vi "CAN Komm.vi"(8 "error in":errorcluster) -> (0 "error out":errorcluster)   [LabVIEW 2020, in "CAN Interface.lvlib"]
uses:
  CAN Interface.lvlib
  CAN Komm Aktionen.ctl
  FGV CAN Daten Aktionen.ctl
  <vilib>/xnet/xnet.llb/XNET CAN Comm State.ctl
  <vilib>/xnet/xnet.llb/XNET Control Scope.ctl
  <vilib>/xnet/xnet.llb/XNET Create Session (Frame Output Stream).vi
  <vilib>/xnet/xnet.llb/XNET Write (Frame CAN).vi
  <vilib>/xnet/xnet.llb/XNET Read (State CAN Comm).vi
  <vilib>/xnet/xnet.llb/XNET Create Session (Frame Input Stream).vi
  <vilib>/xnet/xnet.llb/XNET Read (Frame CAN).vi
  <resource>/objmgr/xnet.rc
  Allgemein/Allgemein.lvlib
panel:
  in  "interface":refnum<k21>="CAN1"
  in  "cluster (:memory:)":refnum<k21>="nixnet_example.CAN_Cluster"
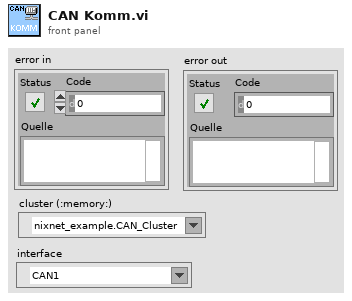
[diagram p1: front panel]
types:
  T1 = typedef "CAN Interface.lvlib/CAN Komm Aktionen.ctl" = enum16{"lesen", "init", "Komm", "beenden", "flush"}
  T2 = typedef "CAN Interface.lvlib/FGV CAN Daten Aktionen.ctl" = enum16{"lesen", "Daten", "Konfig", "laden", "speichern", "Status"}
  T3 = typedef "XNET CAN Comm State.ctl" = u8
  T4 = typedef "CAN Konfig.lvlib/Konfig Daten PC.ctl" = cluster{"Baude Rate":T5, "COM state":u8, "Frame-ID FTIR Start":u32, "Frame-ID FTIR End":u32, "Frame-ID Status Start":u32, "Frame-ID Status End":u32, "Zustand Information":u32, "Aktion":u32, "Frame-ID FTIR Arry":u32[], "Frame-ID Status Arry":u32[], "GPS Start":u32, "Interface":refnum<k21>}
  T5 = typedef "CAN Interface.lvlib/Baude Rate.ctl" = u32
  T6 = typedef "XNET Frame CAN.ctl" = cluster{"timestamp":timestamp, "payload":u8[], "identifier":u32, "type":T7, "extended?":bool, "echo?":bool}
  T7 = typedef "XNET Frame Type CAN.ctl" = u8
  T8 = typedef "XNET Control Scope.ctl" = u32
  T9 = typedef "XNET CAN Comm.ctl" = cluster{"fault code":i32, "fault?":bool, "communication state":T3, "last error":T10, "receive error counter":u8, "transmit error counter":u8, "transceiver error?":bool, "sleep?":bool}
  T10 = typedef "XNET CAN Last Err.ctl" = u8
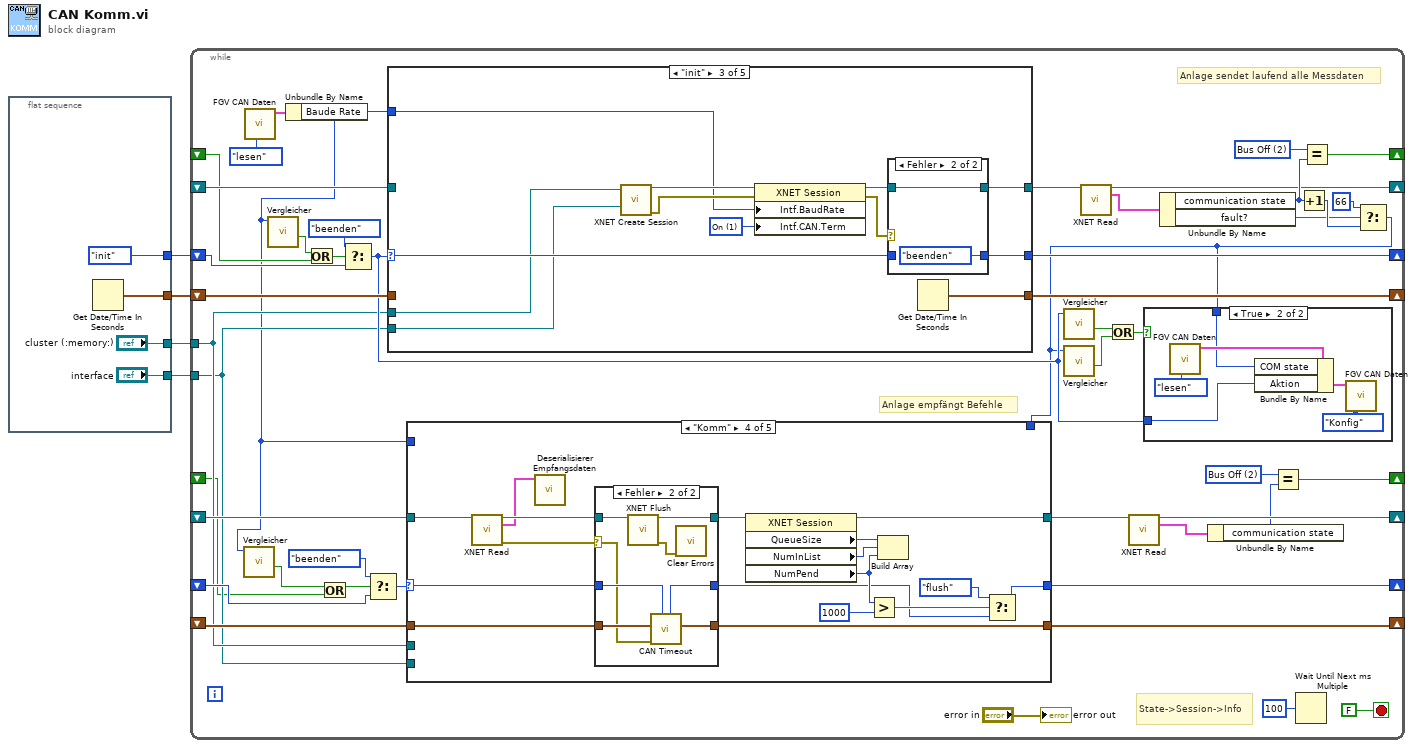
[diagram p0: block diagram]
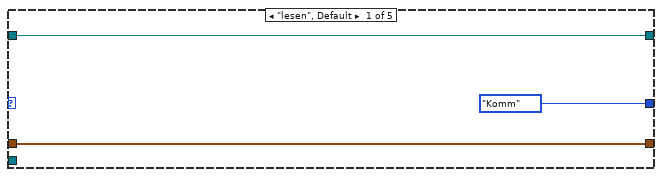
[diagram p3: hidden frame]
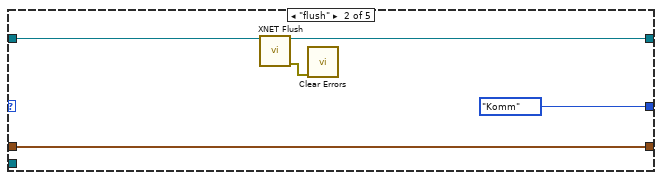
[diagram p4: hidden frame]
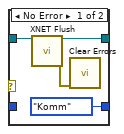
[diagram p5: hidden frame]
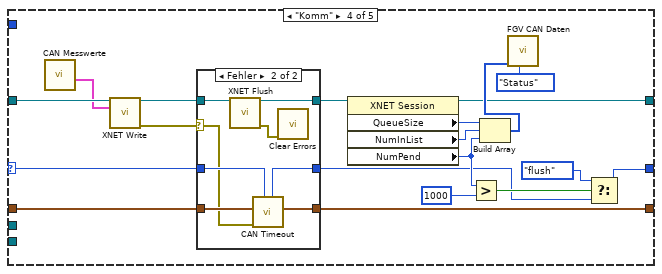
[diagram p6: hidden frame]
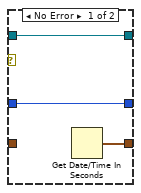
[diagram p7: hidden frame]
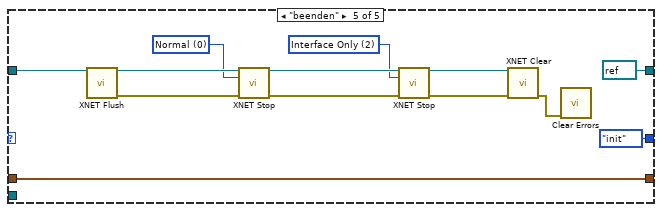
[diagram p8: hidden frame]
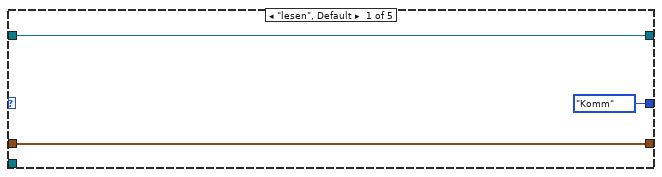
[diagram p9: hidden frame]
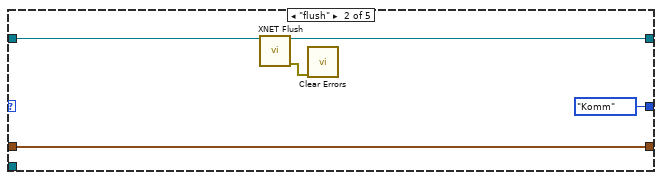
[diagram p10: hidden frame]
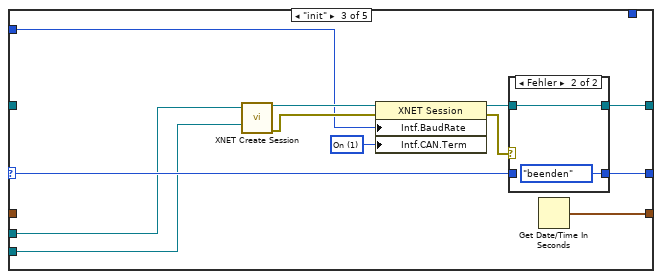
[diagram p11: hidden frame]
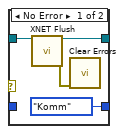
[diagram p12: hidden frame]
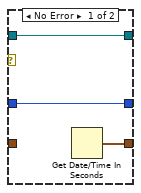
[diagram p13: hidden frame]
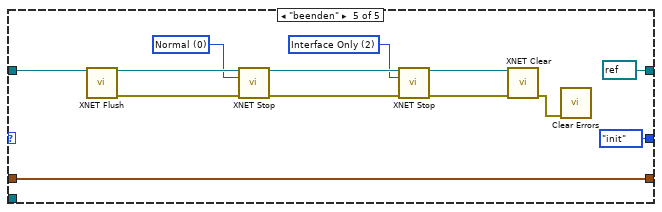
[diagram p14: hidden frame]
diagram:
  n1 = flat-sequence {
    tunnel: [CAN_Komm_Aktionen."init" ("Aktionen")] -> w4
    tunnel: [w7] -> w3
    tunnel: ["cluster (:memory:)"] -> w2
    tunnel: ["interface"] -> w1
    frame #0 {
      n2 = Get Date/Time In Seconds() -> (seconds since 1Jan1904=w7:timestamp)
    }
  }
  n3 = while {
    shift-right: [w14] -> _
    shift-left: _ -> [w55]
    shift-right: [w51] -> _
    shift-left: w4 -> [w48]
    shift-right: [w53] -> _
    shift-left: w3 -> [w54]
    tunnel: w2 -> [w23]
    tunnel: w1 -> [w22]
    shift-right: [w12] -> _
    shift-left: _ -> [w31]
    shift-right: [w20] -> _
    shift-left: _ -> [w28]
    shift-right: [w27] -> _
    shift-left: _ -> [w26]
    shift-right: [w25] -> _
    shift-left: _ -> [w24]
    shift-right: [w13] -> _
    shift-left: _ -> [w15]
    stop <- FALSE stop-if-true
    w18 = T3 2 items=["Error Active", "Error Passive", "Bus Off", "Init"] ("x")
    w33 = T3 2 items=["Error Active", "Error Passive", "Bus Off", "Init"] ("x")
    # "Anlage empfängt Befehle"
    # "Anlage sendet laufend alle Messdaten"
    # "State->Session->Info"
    n4 = call "FGV CAN Daten.vi"("Aktionen"=FGV_CAN_Daten_Aktionen."lesen") -> ("Konfig Daten"=w50:T4)  [unwired: 8 in, 2 out]
    n5 = Unbundle By Name(w50) -> ("Baude Rate"=w10:T5)
    n6 = call "Vergleicher.vi"("Numerisch"=w10) -> ("Änderung"=w30:bool)  [unwired: 10 in]
    n7 = call "Vergleicher.vi"("Numerisch"=w10) -> ("Änderung"=w46:bool)  [unwired: 10 in]
    n8 = Or(x=w46, y=w31) -> (x .or. y?=w32:bool)
    n9 = Or(x=w30, y=w15) -> (x .or. y?=w16:bool)
    n10 = Select(t=CAN_Komm_Aktionen."beenden" ("Aktionen"), s=w32, f=w48) -> (s? t:f=w44:T1)
    n11 = Select(t=CAN_Komm_Aktionen."beenden" ("Aktionen"), s=w16, f=w26) -> (s? t:f=w9:T1)
    n12 = case shown="\"init\"" w44 {
      selector: w44 -> [_ _ w78 w103 _]
      tunnel: w55 -> [w64 w66 _ w106 w128]
      tunnel: [w64 w65 w73 w89 refnum<k21> refnum ("session out")] -> w45
      tunnel: [CAN_Komm_Aktionen."Komm" ("Aktionen") CAN_Komm_Aktionen."Komm" ("Aktionen") w77 w92 CAN_Komm_Aktionen."init" ("Aktionen")] -> w51
      tunnel: w54 -> [w62 w68 _ w104 w129]
      tunnel: [w62 w68 w76 w105 w129] -> w53
      tunnel: w10 -> [_ _ w72 _ _]
      tunnel: w23 -> [_ _ w71 _ _]
      tunnel: w22 -> [_ _ w70 _ _]
      frame "lesen", Default {
      }
      frame "flush" {
        n13 = call <vilib>:"XNET Flush.vi"("session in"=w66) -> ("session out"=w65:refnum<k21>, "error out"=w67:errorcluster)  [unwired: 13 in]
        n14 = call <vilib>:"Clear Errors.vi"("error in (no error)"=w67) -> ()  [unwired: 5 in, 2 out]
      }
      frame "init" {
        w79 = u32 1 items=["Off", "On"] ("Interface:CAN:Termination")
        n15 = call-poly <vilib>:"XNET Create Session.vi"("cluster (:memory:)"=w71, "interface"=w70) -> ("session out"=w80:refnum<k21>, "error out"=w81:errorcluster)  [unwired: 12 in]
        n16 = property class="XNET Session"(reference=w80, error in=w81, "Intf.BaudRate"=w72, "Intf.CAN.Term"=w79) -> (reference out=w74:refnum<k21>, error out=w75:errorcluster)
        n17 = case shown="Fehler" w75 {
          tunnel: w78 -> [_ _]
          tunnel: [CAN_Komm_Aktionen."Komm" ("Aktionen") CAN_Komm_Aktionen."beenden" ("Aktionen")] -> w77
          tunnel: w74 -> [w84 w87]
          tunnel: [w83 w87] -> w73
          frame No Error {
            n18 = call <vilib>:"XNET Flush.vi"("session in"=w84) -> ("session out"=w83:refnum<k21>, "error out"=w82:errorcluster)  [unwired: 13 in]
            n19 = call <vilib>:"Clear Errors.vi"("error in (no error)"=w82) -> ()  [unwired: 5 in, 2 out]
          }
          frame Error {
          }
        }
        n20 = Get Date/Time In Seconds() -> (seconds since 1Jan1904=w76:timestamp)
      }
      frame "Komm" {
        n21 = call "CAN Messwerte.vi"() -> ("CAN data"=w88:T6[])  [unwired: 11 in]
        n22 = call-poly <vilib>:"XNET Write.vi"("session in"=w106, "data"=w88) -> ("session out"=w90:refnum<k21>, "error out"=w102:errorcluster)  [unwired: 1 in, 11 out]
        n23 = case shown="Fehler" w102 {
          selector: w102 -> [_ w113]
          tunnel: [w109 w116] -> w105
          tunnel: w104 -> [_ w117]
          tunnel: w103 -> [w108 w115]
          tunnel: [w108 w114] -> w93
          tunnel: w90 -> [w107 w112]
          tunnel: [w107 w111] -> w101
          frame No Error {
            n24 = Get Date/Time In Seconds() -> (seconds since 1Jan1904=w109:timestamp)
          }
          frame Error {
            n25 = call <vilib>:"XNET Flush.vi"("session in"=w112) -> ("session out"=w111:refnum<k21>, "error out"=w110:errorcluster)  [unwired: 13 in]
            n26 = call "CAN Timeout.vi"("Aktionen"=w115, "Fehler"=w113, "Zeitstempel"=w117) -> ("Zeitstempel"=w116:timestamp, "Aktionen"=w114:T1)  [unwired: 7 in]
            n27 = call <vilib>:"Clear Errors.vi"("error in (no error)"=w110) -> ()  [unwired: 5 in, 2 out]
          }
        }
        n28 = property class="XNET Session"(reference=w101) -> (reference out=w89:refnum<k21>, "QueueSize"=w99:u32, "NumInList"=w98:u32, "NumPend"=w96:u32)  [unwired: 1 in, 1 out]
        n29 = Greater?(x=w96, y=u32 1000) -> (0:w94:bool)
        n30 = Build Array(w99, w98, w96) -> (w97:u32[])
        n31 = call "FGV CAN Daten.vi"("Aktionen"=FGV_CAN_Daten_Aktionen."Status", "Status"=w97) -> ()  [unwired: 7 in, 3 out]
        n32 = Select(t=CAN_Komm_Aktionen."flush", s=w94, f=w93) -> (s? t:f=w92:T1)
      }
      frame "beenden" {
        w121 = T8 2 items=["Normal", "Session Only", "Interface Only", "Session Only Blocking"] ("scope (normal)")
        w124 = T8 0 items=["Normal", "Session Only", "Interface Only", "Session Only Blocking"] ("scope (normal)")
        n33 = call <vilib>:"XNET Flush.vi"("session in"=w128) -> ("session out"=w127:refnum<k21>, "error out"=w126:errorcluster)  [unwired: 13 in]
        n34 = call <vilib>:"XNET Stop.vi"("session in"=w127, "scope (normal)"=w124, "error in (no error)"=w126) -> ("session out"=w123:refnum<k21>, "error out"=w122:errorcluster)  [unwired: 11 in]
        n35 = call <vilib>:"XNET Stop.vi"("session in"=w123, "scope (normal)"=w121, "error in (no error)"=w122) -> ("session out"=w125:refnum<k21>, "error out"=w120:errorcluster)  [unwired: 11 in]
        n36 = call <vilib>:"XNET Clear.vi"("session in"=w125, "error in (no error)"=w120) -> ("error out"=w119:errorcluster)  [unwired: 13 in]
        n37 = call <vilib>:"Clear Errors.vi"("error in (no error)"=w119) -> ()  [unwired: 5 in, 2 out]
      }
    }
    n38 = call "Vergleicher.vi"("Numerisch"=w44) -> ("Änderung"=w41:bool)  [unwired: 10 in]
    n39 = call-poly <vilib>:"XNET Read.vi"("session in"=w45) -> ("session out"=w14:refnum<k21>, "CAN comm"=w43:T9)  [unwired: 12 in, 1 out]
    n40 = Unbundle By Name(w43) -> ("communication state"=w34:T3, "fault?"=w37:bool)
    n41 = Wait Until Next ms Multiple(millisecond multiple=u32 100 ("Vielfache von ms")) -> ()  [unwired: 1 out]
    n42 = Increment(x=w34) -> (x+1=w39:T3)
    n43 = Equal?(x=w33, y=w34) -> (x = y?=w12:bool)
    n44 = Select(t=u8 66, s=w37, f=w39) -> (s? t:f=w11:T3)
    n45 = case shown="\"Komm\"" w9 {
      selector: w9 -> [_ _ w147 w170 _]
      tunnel: w28 -> [w133 w135 _ w173 w195]
      tunnel: [w133 w134 w142 w158 refnum<k21> refnum ("session out")] -> w19
      tunnel: [CAN_Komm_Aktionen."Komm" ("Aktionen") CAN_Komm_Aktionen."Komm" ("Aktionen") w146 w161 CAN_Komm_Aktionen."init" ("Aktionen")] -> w27
      tunnel: w24 -> [w131 w137 _ w171 w196]
      tunnel: [w131 w137 w145 w172 w196] -> w25
      tunnel: w10 -> [_ _ w141 _ _]
      tunnel: w23 -> [_ _ w140 _ _]
      tunnel: w22 -> [_ _ w139 _ _]
      tunnel: w11 -> [_ _ _ _ _]
      frame "lesen", Default {
      }
      frame "flush" {
        n46 = call <vilib>:"XNET Flush.vi"("session in"=w135) -> ("session out"=w134:refnum<k21>, "error out"=w136:errorcluster)  [unwired: 13 in]
        n47 = call <vilib>:"Clear Errors.vi"("error in (no error)"=w136) -> ()  [unwired: 5 in, 2 out]
      }
      frame "init" {
        w148 = u32 1 items=["Off", "On"] ("Interface:CAN:Termination")
        n48 = call-poly <vilib>:"XNET Create Session.vi"("cluster (:memory:)"=w140, "interface"=w139) -> ("session out"=w149:refnum<k21>, "error out"=w150:errorcluster)  [unwired: 12 in]
        n49 = property class="XNET Session"(reference=w149, error in=w150, "Intf.BaudRate"=w141, "Intf.CAN.Term"=w148) -> (reference out=w143:refnum<k21>, error out=w144:errorcluster)
        n50 = case shown="Fehler" w144 {
          tunnel: w147 -> [_ _]
          tunnel: [CAN_Komm_Aktionen."Komm" ("Aktionen") CAN_Komm_Aktionen."beenden" ("Aktionen")] -> w146
          tunnel: w143 -> [w153 w156]
          tunnel: [w152 w156] -> w142
          frame No Error {
            n51 = call <vilib>:"XNET Flush.vi"("session in"=w153) -> ("session out"=w152:refnum<k21>, "error out"=w151:errorcluster)  [unwired: 13 in]
            n52 = call <vilib>:"Clear Errors.vi"("error in (no error)"=w151) -> ()  [unwired: 5 in, 2 out]
          }
          frame Error {
          }
        }
        n53 = Get Date/Time In Seconds() -> (seconds since 1Jan1904=w145:timestamp)
      }
      frame "Komm" {
        n54 = call-poly <vilib>:"XNET Read.vi"("session in"=w173) -> ("session out"=w159:refnum<k21>, "data"=w157:T6[], "error out"=w169:errorcluster)  [unwired: 11 in, 1 out]
        n55 = call "Deserialisierer Empfangsdaten.vi"("CAN Daten"=w157) -> ()  [unwired: 11 in]
        n56 = case shown="Fehler" w169 {
          selector: w169 -> [_ w180]
          tunnel: [w176 w183] -> w172
          tunnel: w171 -> [_ w184]
          tunnel: w170 -> [w175 w182]
          tunnel: [w175 w181] -> w162
          tunnel: w159 -> [w174 w179]
          tunnel: [w174 w178] -> w168
          frame No Error {
            n57 = Get Date/Time In Seconds() -> (seconds since 1Jan1904=w176:timestamp)
          }
          frame Error {
            n58 = call <vilib>:"XNET Flush.vi"("session in"=w179) -> ("session out"=w178:refnum<k21>, "error out"=w177:errorcluster)  [unwired: 13 in]
            n59 = call "CAN Timeout.vi"("Aktionen"=w182, "Fehler"=w180, "Zeitstempel"=w184) -> ("Zeitstempel"=w183:timestamp, "Aktionen"=w181:T1)  [unwired: 7 in]
            n60 = call <vilib>:"Clear Errors.vi"("error in (no error)"=w177) -> ()  [unwired: 5 in, 2 out]
          }
        }
        n61 = property class="XNET Session"(reference=w168) -> (reference out=w158:refnum<k21>, "QueueSize"=w167:u32, "NumInList"=w166:u32, "NumPend"=w165:u32)  [unwired: 1 in, 1 out]
        n62 = Greater?(x=w165, y=u32 1000) -> (0:w163:bool)
        n63 = Build Array(w167, w166, w165) -> ()  [unwired: 1 out]
        n64 = Select(t=CAN_Komm_Aktionen."flush", s=w163, f=w162) -> (s? t:f=w161:T1)
      }
      frame "beenden" {
        w188 = T8 2 items=["Normal", "Session Only", "Interface Only", "Session Only Blocking"] ("scope (normal)")
        w191 = T8 0 items=["Normal", "Session Only", "Interface Only", "Session Only Blocking"] ("scope (normal)")
        n65 = call <vilib>:"XNET Flush.vi"("session in"=w195) -> ("session out"=w194:refnum<k21>, "error out"=w193:errorcluster)  [unwired: 13 in]
        n66 = call <vilib>:"XNET Stop.vi"("session in"=w194, "scope (normal)"=w191, "error in (no error)"=w193) -> ("session out"=w190:refnum<k21>, "error out"=w189:errorcluster)  [unwired: 11 in]
        n67 = call <vilib>:"XNET Stop.vi"("session in"=w190, "scope (normal)"=w188, "error in (no error)"=w189) -> ("session out"=w192:refnum<k21>, "error out"=w187:errorcluster)  [unwired: 11 in]
        n68 = call <vilib>:"XNET Clear.vi"("session in"=w192, "error in (no error)"=w187) -> ("error out"=w186:errorcluster)  [unwired: 13 in]
        n69 = call <vilib>:"Clear Errors.vi"("error in (no error)"=w186) -> ()  [unwired: 5 in, 2 out]
      }
    }
    n70 = call "Vergleicher.vi"("Numerisch"=w11) -> ("Änderung"=w40:bool)  [unwired: 10 in]
    n71 = Or(x=w41, y=w40) -> (x .or. y?=w42:bool)
    n72 = call-poly <vilib>:"XNET Read.vi"("session in"=w19) -> ("session out"=w20:refnum<k21>, "CAN comm"=w21:T9)  [unwired: 12 in, 1 out]
    n73 = case shown="True" w42 {
      tunnel: w44 -> [_ w61]
      tunnel: w11 -> [_ w56]
      frame False {
      }
      frame True {
        n74 = call "FGV CAN Daten.vi"("Aktionen"=FGV_CAN_Daten_Aktionen."lesen") -> ("Konfig Daten"=w57:T4)  [unwired: 8 in, 2 out]
        n75 = Bundle By Name(cluster=w57, "COM state"=w56, "Aktion"=w61) -> (w59:T4)
        n76 = call "FGV CAN Daten.vi"("Aktionen"=FGV_CAN_Daten_Aktionen."Konfig", "Konfig Daten 2"=w59) -> ()  [unwired: 7 in, 3 out]
      }
    }
    n77 = Unbundle By Name(w21) -> ("communication state"=w17:T3)
    n78 = Equal?(x=w18, y=w17) -> (x = y?=w13:bool)
    "error out" <- "error in"
  }
